vi "Actor.vi"(4 "Creator":refnum<user-event>, 6 "Creator Alias":string, 8 "Self Alias":string, 9 "Queue of Self":refnum<queue>, 10 "jettl":refnum<class "jettl.lvclass">) -> ()   [LabVIEW 2021, in "jettl.lvlib" / "Base Event.lvlib" / "Base Event.lvclass"]
uses:
  Base Event.lvclass
  Base Event.lvclass/Base Event.ctl
  Last Ack Created Msg Strategy/Last Ack Created Msg Strategy.lvlib
  jettl/jettl.lvclass
  Addresses Strategy/Addresses Strategy.lvlib
  Last Ack Creator Msg Strategy/Last Ack Creator Msg Strategy.lvlib
  C:/git/jettl/jettl/jettl/jettl/jettl.lvclass
  C:/git/jettl/jettl/Merge Error Msg Strategy/Merge Error/Merge Error.lvclass
  Msg Strategy/Msg Strategy.lvclass
  C:/git/jettl/jettl/jettl/Base Event/Base Event/Base Event.lvclass
  C:/git/jettl/jettl/Create Msg Strategy/Create/Create.lvclass
  C:/git/jettl/jettl/jettl/Last Ack Created Msg Strategy/Last Ack Created/Last Ack Created.lvclass
  C:/git/jettl/jettl/jettl/Last Ack Creator Msg Strategy/Last Ack Creator/Last Ack Creator.lvclass
  C:/git/jettl/jettl/Override Error Msg Strategy/Override Error/Override Error.lvclass
  C:/git/jettl/jettl/Setup Msg Strategy/Setup/Setup.lvclass
  C:/git/jettl/jettl/Teardown Msg Strategy/Teardown/Teardown.lvclass
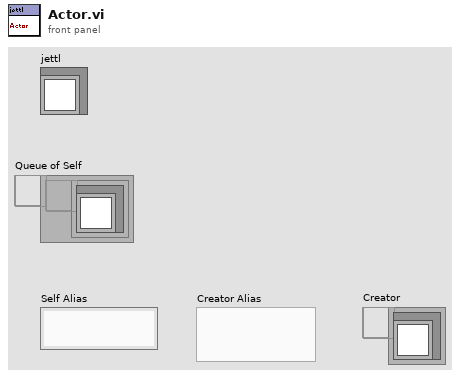
[diagram p1: front panel]
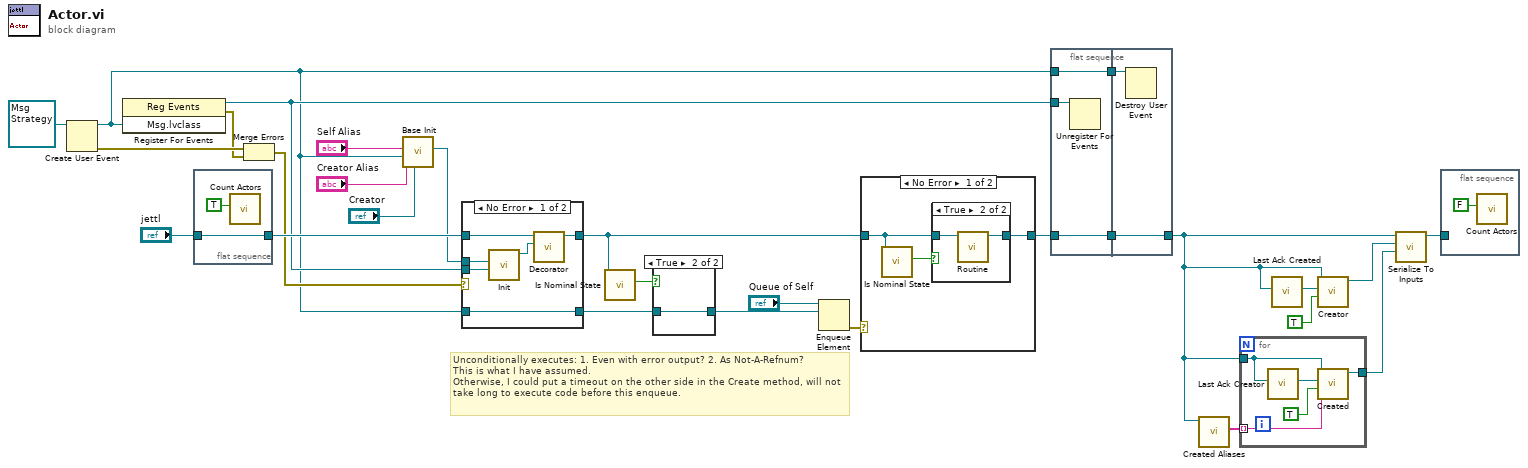
[diagram p0: block diagram]
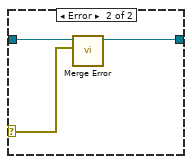
[diagram p3: hidden frame]
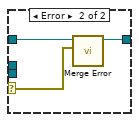
[diagram p5: hidden frame]
diagram:
  # "Unconditionally executes: 1. Even with error output? 2. As Not-A-Refnum?\nThis is what I have assumed.\nOtherwise, I could put a timeout on the other side in the Create method, will not take long to execute code before this enqueue."
  n1 = Create User Event(user event datatype=refnum<class "Msg Strategy.lvclass"> refnum ("Msg.lvclass")) -> (user event=w4:refnum<user-event>, error out=w11:errorcluster)  [unwired: 1 in]
  n2 = register-events(w4) -> (reference out=w7:refnum<event-registration>, error out=w9:errorcluster)  [unwired: 2 in]
  n3 = flat-sequence {
    tunnel: [w29] -> w28
    tunnel: "jettl" -> [w29]
    frame #0 {
      n4 = call "Count Actors.vi"("Increment?"=TRUE) -> ()  [unwired: 11 in]
    }
  }
  n5 = Merge Errors(w11, w9) -> (w8:errorcluster)
  n6 = call "Base Init.vi"("Creator"="Creator", "Creator Alias"="Creator Alias", "Self"=w4, "Self Alias"="Self Alias") -> ("Addresses Strategy out"=w19:refnum<class "Addresses Strategy.lvclass">)  [unwired: 7 in]
  n7 = case shown="No Error" w8 {
    selector: w8 -> [_ w38]
    tunnel: [w35 w39] -> w24
    tunnel: w28 -> [w34 w37]
    tunnel: w4 -> [w36 _]
    tunnel: [w36 _] -> w26
    tunnel: w19 -> [w32 _]
    tunnel: w7 -> [w31 _]
    frame No Error {
      n8 = call "Init.vi"("Register"=w31, "Addresses Strategy"=w32) -> ("Base Event out"=w33:refnum<class "Base Event.lvclass">)  [unwired: 9 in]
      n9 = call-dynamic "Decorator.vi"("jettl"=w33, "jettl in"=w34) -> ("jettl out"=w35:refnum<class "jettl.lvclass">)  [unwired: 9 in]
    }
    frame Error {
      n10 = call-dynamic "Merge Error.vi"("Error"=w38, "Merge Error in"=w37) -> ("Merge Error out"=w39:refnum<class "jettl.lvclass">)  [unwired: 9 in]
    }
  }
  n11 = call-dynamic "Is Nominal State.vi"("jettl in"=w24) -> ("Is Nominal State?"=w25:bool)  [unwired: 10 in]
  n12 = case shown="True" w25 {
    tunnel: [_ w40] -> w2
    tunnel: w26 -> [_ w40]
    frame False {
    }
    frame True {
    }
  }
  n13 = Enqueue Element(queue="Queue of Self", element=w2) -> (error out=w23:errorcluster)  [unwired: 2 in, 2 out]
  n14 = case shown="No Error" w23 {
    selector: w23 -> [_ w47]
    tunnel: [w43 w48] -> w27
    tunnel: w24 -> [w41 w49]
    frame No Error {
      n15 = call-dynamic "Is Nominal State.vi"("jettl in"=w41) -> ("Is Nominal State?"=w42:bool)  [unwired: 10 in]
      n16 = case shown="True" w42 {
        tunnel: w41 -> [w44 w46]
        tunnel: [w44 w45] -> w43
        frame False {
        }
        frame True {
          n17 = call-dynamic "Routine.vi"("jettl in"=w46) -> ("jettl out"=w45:refnum<class "jettl.lvclass">)  [unwired: 10 in]
        }
      }
    }
    frame Error {
      n18 = call-dynamic "Merge Error.vi"("Error"=w47, "Merge Error in"=w49) -> ("Merge Error out"=w48:refnum<class "jettl.lvclass">)  [unwired: 9 in]
    }
  }
  n19 = flat-sequence {
    tunnel: w4 -> [w50]
    tunnel: w27 -> [w52]
    tunnel: w7 -> [w51]
    tunnel: [w52] -> w6
    tunnel: [w50] -> w5
    tunnel: [w54] -> w12
    tunnel: w6 -> [w54]
    tunnel: w5 -> [w53]
    frame #0 {
      n20 = Unregister For Events(event registration refnum=w51) -> ()  [unwired: 1 in, 1 out]
    }
    frame #1 {
      n21 = Destroy User Event(user event=w53) -> ()  [unwired: 1 in, 1 out]
    }
  }
  n22 = call-dynamic "Created Aliases.vi"("jettl in"=w12) -> ("Created Aliases"=w16:string[])  [unwired: 9 in, 1 out]
  n23 = for {
    tunnel: w12 -> [w56]
    tunnel: w16 -> [w59] mode=indexing
    tunnel: [w55] -> w14
    n24 = call "Last Ack Creator.vi"("jettl"=w56) -> ("Msg Strategy"=w57:refnum<class "Msg Strategy.lvclass">)  [unwired: 10 in]
    n25 = call-dynamic "Created.vi"("Created Alias"=w59, "Priority?"=TRUE, "Msg Strategy"=w57, "jettl in"=w56) -> ("jettl out"=w55:refnum<class "jettl.lvclass">)  [unwired: 7 in]
  }
  n26 = call "Last Ack Created.vi"("jettl"=w12) -> ("Msg Strategy"=w18:refnum<class "Msg Strategy.lvclass">)  [unwired: 10 in]
  n27 = call-dynamic "Creator.vi"("Priority?"=TRUE, "Msg Strategy"=w18, "jettl in"=w12) -> ("jettl out"=w15:refnum<class "jettl.lvclass">)  [unwired: 8 in]
  n28 = call-dynamic "Serialize To Inputs.vi"("Input 2"=w14, "Input 1"=w15, "jettl in"=w12) -> ("jettl out"=w13:refnum<class "jettl.lvclass">)  [unwired: 8 in]
  n29 = flat-sequence {
    tunnel: w13 -> [_]
    frame #0 {
      n30 = call "Count Actors.vi"("Increment?"=FALSE) -> ()  [unwired: 11 in]
    }
  }
